vi "TSC Material Theme Mode--constant.vi"() -> (3 "Theme Path Tag":string)   [LabVIEW 2021]
doc: "CONSTANT VI - defines the user VI tag for the theme mode\n\n<b>Code Developed By:</b>\nDaniel Coons\nTechnology Service Corporation\nwww.tsc.com/atcs"
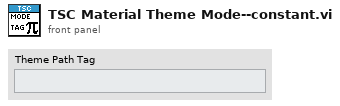
[diagram p1: front panel]
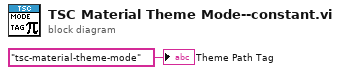
[diagram p0: block diagram]
diagram:
  "Theme Path Tag" <- "tsc-material-theme-mode" ("Theme Path Tag")
